vi "BuoyIdentifier.vi"(1 "Y Pixel":i32, 2 "X Pixel":i32) -> (0 "Buoy Selector":i32(listbox))   [LabVIEW 2012]
panel:
  out "D":bool
  out "C":bool
  out "B":bool
  out "A":bool
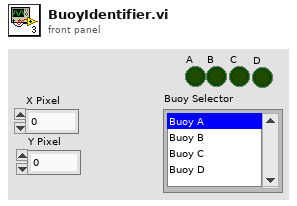
[diagram p1: front panel]
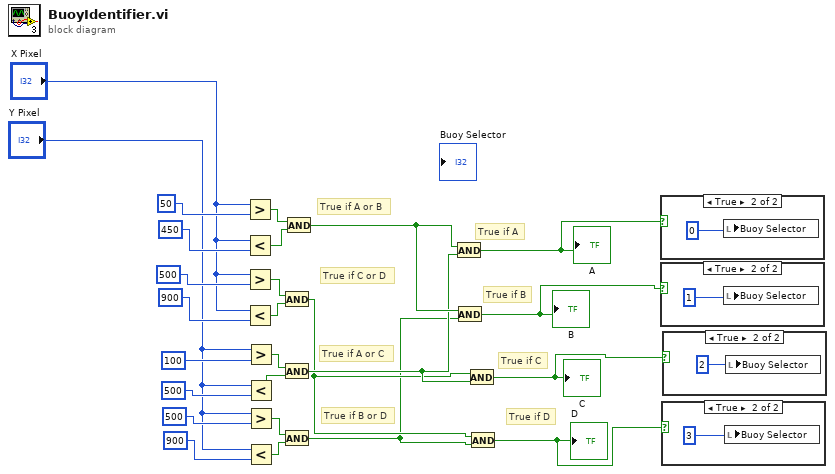
[diagram p0: block diagram]
diagram:
  # "True if D"
  # "True if C"
  # "True if B"
  # "True if A"
  # "True if B or D"
  # "True if A or C"
  # "True if C or D"
  # "True if A or B"
  n1 = Greater?(x="X Pixel", y=50) -> (0:w18:bool)
  n2 = Less?(x="X Pixel", y=450) -> (x < y?=w17:bool)
  n3 = Greater?(x="X Pixel", y=500) -> (0:w16:bool)
  n4 = Less?(x="X Pixel", y=900) -> (x < y?=w15:bool)
  n5 = Greater?(x="Y Pixel", y=100) -> (0:w14:bool)
  n6 = Less?(x="Y Pixel", y=500) -> (x < y?=w13:bool)
  n7 = Greater?(x="Y Pixel", y=500) -> (0:w12:bool)
  n8 = Less?(x="Y Pixel", y=900) -> (x < y?=w11:bool)
  n9 = And(x=w16, y=w15) -> (x .and. y?=w8:bool)
  n10 = And(x=w14, y=w13) -> (x .and. y?=w9:bool)
  n11 = And(x=w12, y=w11) -> (x .and. y?=w7:bool)
  n12 = And(x=w18, y=w17) -> (x .and. y?=w10:bool)
  n13 = And(x=w10, y=w9) -> (x .and. y?=w6:bool)
  "A" <- w6
  n14 = And(x=w10, y=w7) -> (x .and. y?=w5:bool)
  "B" <- w5
  n15 = And(x=w8, y=w9) -> (x .and. y?=w4:bool)
  "C" <- w4
  n16 = And(x=w8, y=w7) -> (x .and. y?=w3:bool)
  "D" <- w3
  n17 = case shown="True" w6 {
    frame False {
    }
    frame True {
      n18 = local write "Buoy Selector"(0 ("Listbox")) -> ()
    }
  }
  n19 = case shown="True" w5 {
    frame False {
    }
    frame True {
      n20 = local write "Buoy Selector"(1 ("Listbox")) -> ()
    }
  }
  n21 = case shown="True" w3 {
    frame False {
    }
    frame True {
      n22 = local write "Buoy Selector"(3 ("Listbox")) -> ()
    }
  }
  n23 = case shown="True" w4 {
    frame False {
    }
    frame True {
      n24 = local write "Buoy Selector"(2 ("Listbox")) -> ()
    }
  }
